vi "reset port-odor ring value (sub-vi).vi"(8 "error in (no error)":errorcluster, 10 "reset value (off)":T1 items=["off"], 11 "port-odor ring refnum":refnum<vi>) -> (0 "error out":errorcluster, 3 "port-odor ring refnum out":refnum<vi>)   [LabVIEW 2021]
uses:
  type-defs/port-odor ring (type def).ctl
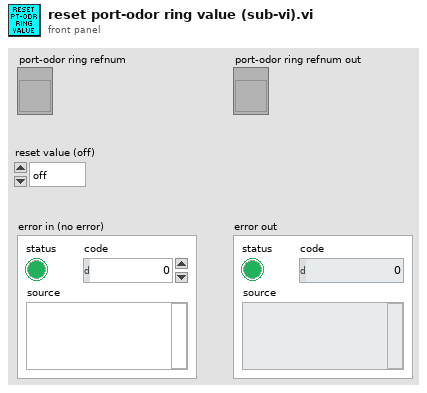
[diagram p1: front panel]
types:
  T1 = typedef "port-odor ring (type def).ctl" = u16
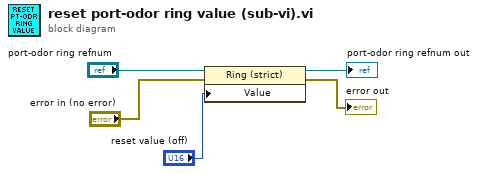
[diagram p0: block diagram]
diagram:
  n1 = property class="Ring (strict)"(reference="port-odor ring refnum", error in="error in (no error)", "Value"="reset value (off)") -> (reference out=→"port-odor ring refnum out":refnum<vi>, error out=→"error out":errorcluster)
